vi "Read hkParam.vi"(8 "error in":errorcluster, 11 "CRDS Cell Data in":refnum<class "CRDS Cell Data.lvclass">) -> (0 "error out":errorcluster, 2 "hkParam":T1={"rhDilFac"=1.0, "Q"=0.0, "Tmean"=0.0, "extDilFac"=1.0, "rhCell"=0.0, "P"=0.0, "T"=0.0}, 3 "CRDS Cell Data out":refnum<class "CRDS Cell Data.lvclass">)   [LabVIEW 2015, in "CRDS Cell Data.lvclass"]
uses:
  CRDS Cell Data.lvclass
  calData.ctl
  CRDS Cell Data.lvclass/CRDS Cell Data.ctl
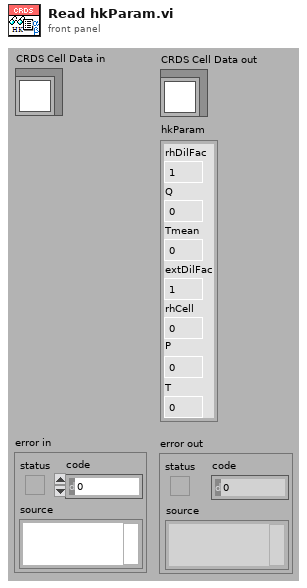
[diagram p1: front panel]
types:
  T1 = typedef "calData.ctl" = cluster{"rhDilFac":sgl, "Q":sgl, "Tmean":sgl, "extDilFac":sgl, "rhCell":sgl, "P":sgl, "T":sgl}
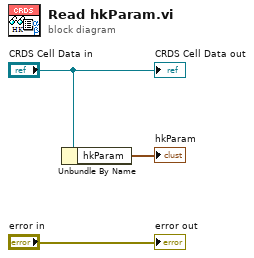
[diagram p0: block diagram]
diagram:
  n1 = Unbundle By Name("CRDS Cell Data in") -> ("hkParam"=→"hkParam":T1)
  "error out" <- "error in"
  "CRDS Cell Data out" <- "CRDS Cell Data in"
